vi "Select Worksheet by Index.vi"(2 "error in (no error)":errorcluster, 3 "Worksheet Index":dbl, 4 "Report Ref In":T1) -> (0 "error out":errorcluster, 1 "Report Ref Out":T1)   [LabVIEW 2026, in "XCel Report Engine.lvlib"]
uses:
  XCel Report Engine.lvlib
  Controls/Report Ref.ctl
  C:/Users/m.santucci/Documents/ChatGPT/LV_REPORT_ENGINE/.net/src/XCelReportEngine/bin/Release/net48/XCelReportEngine.dll
  .net/src/XCelReportEngine/bin/Release/net48/XCelReportEngine.dll
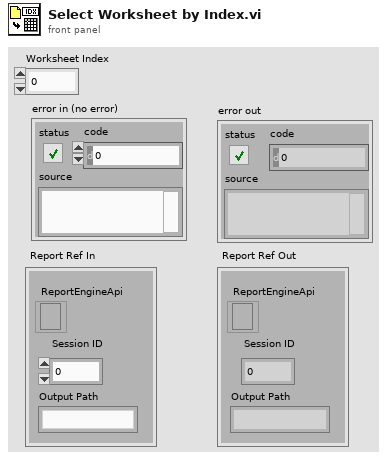
[diagram p1: front panel]
types:
  T1 = typedef "XCel Report Engine.lvlib/Report Ref.ctl" = cluster{"Session ID":i32, "Output Path":string, "ReportEngineApi":refnum<k24>}
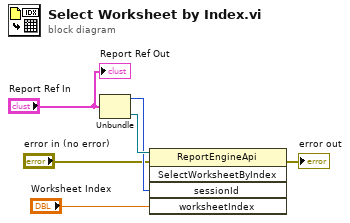
[diagram p0: block diagram]
diagram:
  n1 = Unbundle("Report Ref In") -> ("Session ID"=w4:i32, "ReportEngineApi"=w5:refnum<k24>)  [unwired: 1 out]
  n2 = invoke class="ReportEngineApi" method="SelectWorksheetByIndex"(reference=w5, error in="error in (no error)", "sessionId"=w4, "worksheetIndex"="Worksheet Index") -> (error out=→"error out":errorcluster)  [unwired: 1 in, 4 out]
  "Report Ref Out" <- "Report Ref In"
